vi "Retrieve Full Scale.vi"(8 "error in":errorcluster, 10 "Model Data":string, 11 "Alicat Device in":refnum<class "Alicat Device.lvclass">) -> (0 "error out":errorcluster, 1 "Type":string, 2 "Full Scale":sgl, 3 "Alicat Device out":refnum<class "Alicat Device.lvclass">, 4 "ModelOut":string)   [LabVIEW 2015, in "Alicat Lib.lvlib" / "Alicat Device.lvclass"]
doc: "The full scale of the device defines the input command for the setpoint (if the device is a controller). The setpoint command will use the full scale (FS) such that \n\nVal = SP*64000/FS"
uses:
  Alicat Device.lvclass
  <vilib>/MSR Consulting, LLC/Configurable Device/Configurable Device.lvclass/Configurable Device.ctl
  Alicat Device.lvclass/Alicat Device.ctl
  <vilib>/MSR Consulting, LLC/Configurable Device/Accessors/Write Model.vi
  <vilib>/MSR Consulting, LLC/Configurable Device/Accessors/Write SN.vi
  <vilib>/NI/Tools/String/Tools_String.lvlib
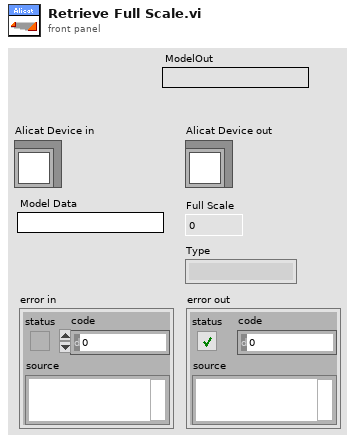
[diagram p1: front panel]
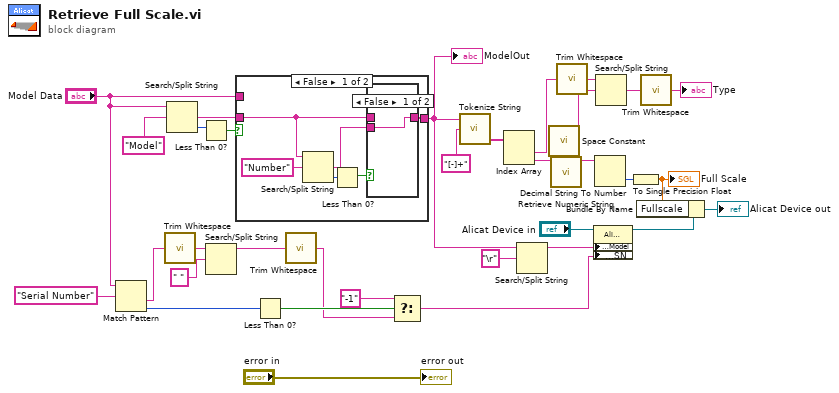
[diagram p0: block diagram]
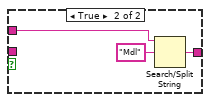
[diagram p3: hidden frame]
diagram:
  n1 = Match Pattern(string="Model Data", regular expression="Serial Number" ("search string/char (-)")) -> (after substring=w2:string, offset past match=w11:i32)  [unwired: 1 in, 2 out]
  n2 = call <vilib>:"Trim Whitespace.vi"("string"=w2) -> ("trimmed string"=w1:string)  [unwired: 1 in]
  n3 = Search/Split String(string="Model Data", search string/char (-)="Model") -> (match + rest of string=w17:string, offset of match=w19:i32)  [unwired: 1 in, 1 out]
  n4 = Less Than 0?(x=w19) -> (x < 0?=w18:bool)
  n5 = Search/Split String(string=w1, search string/char (-)=" ") -> (substring before match=w10:string)  [unwired: 1 in, 2 out]
  n6 = case shown="False" w18 {
    tunnel: "Model Data" -> [_ w44]
    tunnel: w17 -> [w36 _]
    tunnel: [w35 w42] -> w5
    frame False {
      n7 = Search/Split String(string=w36, search string/char (-)="Number") -> (match + rest of string=w34:string, offset of match=w38:i32)  [unwired: 1 in, 1 out]
      n8 = Less Than 0?(x=w38) -> (x < 0?=w37:bool)
      n9 = case shown="False" w37 {
        tunnel: w36 -> [_ w41]
        tunnel: [w40 w41] -> w35
        tunnel: w34 -> [w40 _]
        frame False {
        }
        frame True {
        }
      }
    }
    frame True {
      n10 = Search/Split String(string=w44, search string/char (-)="Mdl") -> (match + rest of string=w42:string)  [unwired: 1 in, 2 out]
    }
  }
  "ModelOut" <- w5
  n11 = Less Than 0?(x=w11) -> (x < 0?=w14:bool)
  n12 = call <vilib>:"Trim Whitespace.vi"("string"=w10) -> ("trimmed string"=w9:string)  [unwired: 1 in]
  n13 = Select(t="-1", s=w14, f=w9) -> (s? t:f=w7:string)
  n14 = call <vilib>:"Tokenize String.vi"("delimiter ([\\s\\t\\n\\r]+)"="[-]+" ("delimiter ([\\s\\t\\n\\r]+)"), "input string"=w5) -> ("token array"=w32:string[])  [unwired: 2 in, 1 out]
  n15 = Index Array(array=w32) -> (element #1=w28:string, element #2=w29:string)  [unwired: 2 in]
  n16 = Search/Split String(string=w5, search string/char (-)="\r") -> (substring before match=w4:string)  [unwired: 1 in, 2 out]
  n17 = call <vilib>:"Space Constant.vi"() -> ("String"=w26:string)
  n18 = call <vilib>:"Retrieve Numeric String.vi"("String in"=w29) -> ("Numeric String"=w31:string)  [unwired: 10 in]
  n19 = call <vilib>:"Trim Whitespace.vi"("string"=w28) -> ("trimmed string"=w27:string)  [unwired: 1 in]
  n20 = property class="Alicat Device"(reference="Alicat Device in", "Accessors:Model"=w4, "Accessors:SN"=w7) -> (reference out=w15:refnum<class "Alicat Device.lvclass">)  [unwired: 1 in, 1 out]
  n21 = Decimal String To Number(string=w31) -> (number=w30:i32)  [unwired: 2 in, 1 out]
  n22 = Search/Split String(string=w27, search string/char (-)=w26) -> (match + rest of string=w25:string)  [unwired: 1 in, 2 out]
  n23 = To Single Precision Float(number=w30) -> (single precision float=w23:sgl)
  "Full Scale" <- w23
  n24 = Bundle By Name(cluster=w15, "Fullscale"=w23) -> (→"Alicat Device out":refnum<class "Alicat Device.lvclass">)
  n25 = call <vilib>:"Trim Whitespace.vi"("string"=w25) -> ("trimmed string"=→"Type":string)  [unwired: 1 in]
  "error out" <- "error in"
